vi "CloseDevice.vi"(8 "error in (no error)":errorcluster caption="错误输入（无错误）", 10 "DeviceInd":u32, 11 "type":u16(ring)=2 items=["USB-CAN"=2, "USB-CAN2.0"=3]) -> (0 "error out":errorcluster caption="错误输出", 3 "success":bool)   [LabVIEW 2011]
uses:
  data/ControlCAN.dll
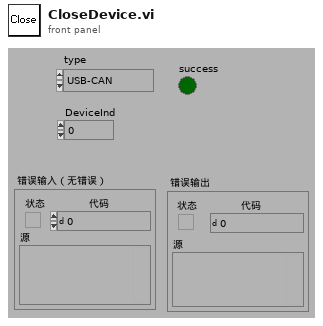
[diagram p1: front panel]
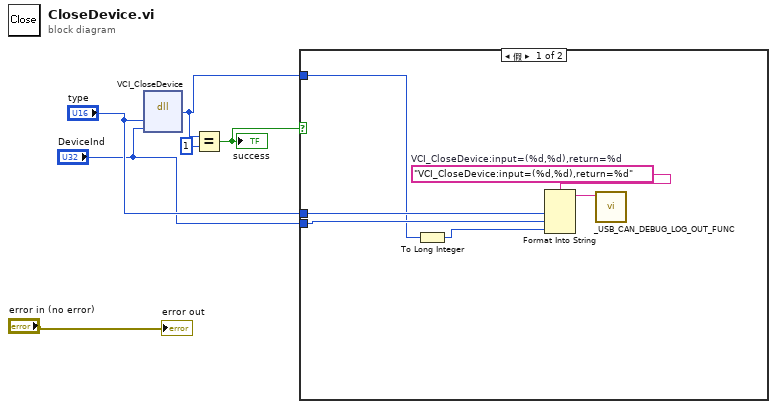
[diagram p0: block diagram]
diagram:
  n1 = dll-call lib="PTH1Mabs ZHost_E工作TnewcodeUSB CAN Tool1.98dataControlCAN.dll" fn="VCI_CloseDevice"("DeviceType"="type", "DeviceInd"="DeviceInd") -> ("返回类型"=w1:u32)  [unwired: 5 in, 2 out]
  n2 = Equal?(x=w1, y=u32 1) -> (x = y?=w4:bool)
  "success" <- w4
  n3 = case shown="假" w4 {
    tunnel: "type" -> [w11 _]
    tunnel: "DeviceInd" -> [w10 _]
    tunnel: w1 -> [w8 _]
    frame False {
      w7 = "VCI_CloseDevice:input=(%d,%d),return=%d"  # VCI_CloseDevice:input=(%d,%d),return=%d
      n4 = To Long Integer(number=w8) -> (32bit integer=w9:i32)
      n5 = Format Into String(format string=w7, w11, w10, w9) -> (resulting string=w12:string)  [unwired: 2 in, 1 out]
      n6 = call "_USB_CAN_DEBUG_LOG_OUT_FUNC.vi"("Info"=w12) -> ()  [unwired: 11 in]
    }
    frame True {
    }
  }
  "error out" <- "error in (no error)"
